vi "failUnlessError.vi"(8 "error in (no error)":errorcluster, 10 "error":errorcluster, 11 "TestCase in":refnum<class "TestCase.lvclass">) -> (0 "error out":errorcluster, 3 "TestCase out":refnum<class "TestCase.lvclass">)   [LabVIEW 2011, in "TestCase.lvclass"]
doc: "{Obsolete - kept for compatiblity only}\n\nFail if 'error.status'=FALSE. 'error' is the error generated by the task. 'task' is the description of the task failure. 'error in' is for framework errors not related to the test task."
uses:
  TestCase.lvclass
panel:
  in  "task (\"\")":string
  # "JKI VI Tester for LabVIEW\nhttp://jkisoft.com/vi-tester\nCopyright (C) 2007-2009, JKI <info@jkisoft.com>\nALL RIGHTS RESERVED"
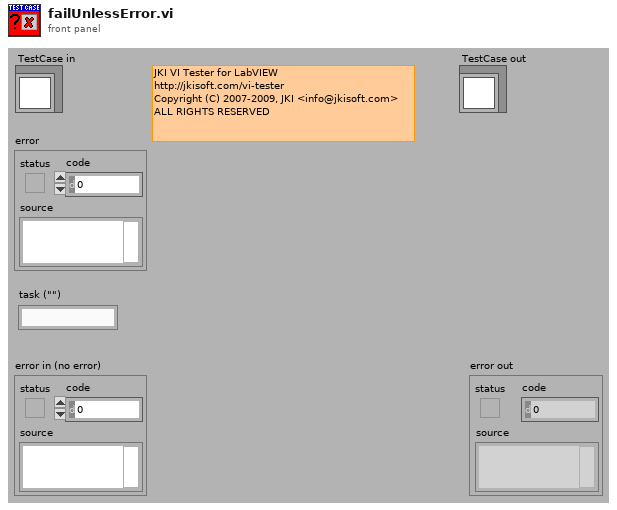
[diagram p1: front panel]
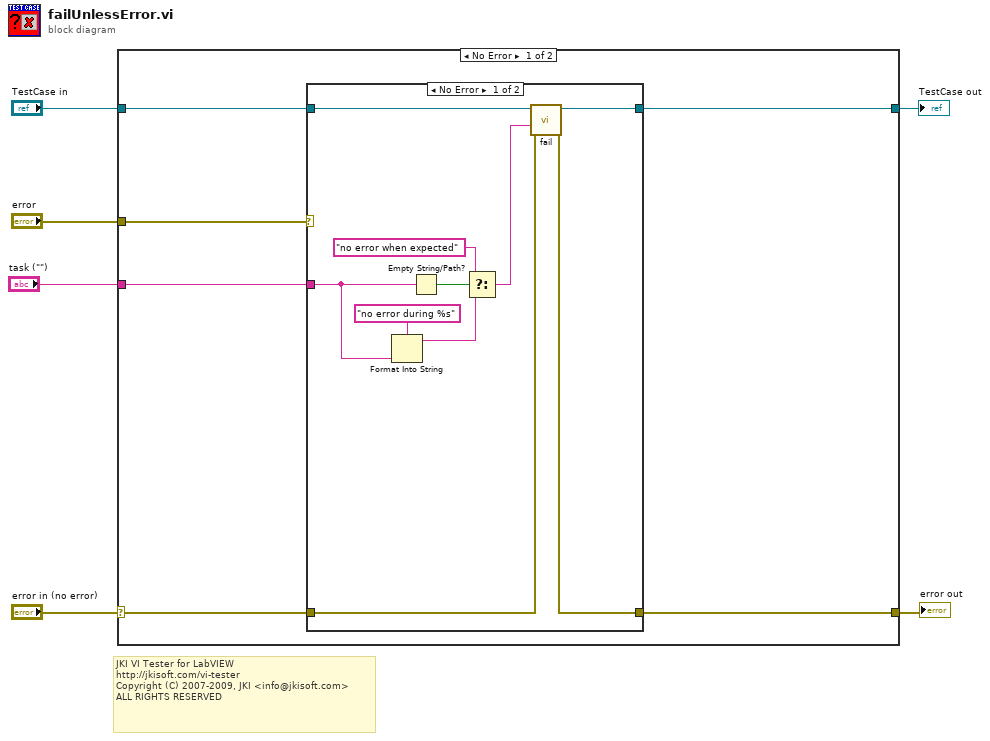
[diagram p0: block diagram]
diagram:
  # "JKI VI Tester for LabVIEW\nhttp://jkisoft.com/vi-tester\nCopyright (C) 2007-2009, JKI <info@jkisoft.com>\nALL RIGHTS RESERVED"
  n1 = case shown="No Error" "error in (no error)" {
    selector: "error in (no error)" -> [w11 w26]
    tunnel: [w10 w26] -> w5
    tunnel: [w8 w25] -> w3
    tunnel: "TestCase in" -> [w9 w25]
    tunnel: "error" -> [w12 _]
    tunnel: "task (\"\")" -> [w7 _]
    frame No Error {
      n2 = case shown="No Error" w12 {
        tunnel: [w21 w24] -> w10
        tunnel: w11 -> [w22 w24]
        tunnel: w9 -> [w20 w23]
        tunnel: [w19 w23] -> w8
        tunnel: w7 -> [w17 _]
        frame No Error {
          n3 = Format Into String(format string="no error during %s", w17) -> (resulting string=w13:string)  [unwired: 2 in, 1 out]
          n4 = Empty String/Path?(string/path=w17) -> (empty?=w16:bool)
          n5 = Select(t="no error when expected" ("message (\"\")"), s=w16, f=w13) -> (s? t:f=w14:string)
          n6 = call-dynamic "fail.vi"("error in (no error)"=w22, "message (\"\")"=w14, "TestCase in"=w20) -> ("error out"=w21:errorcluster, "TestCase out"=w19:refnum<class "TestCase.lvclass">)  [unwired: 7 in]
        }
        frame Error {
        }
      }
    }
    frame Error {
    }
  }
  "error out" <- w5
  "TestCase out" <- w3
